vi "CALCULADORA SIRSA.vi"() -> ()   [LabVIEW 2018]
panel:
  out "accion":bool
  out "años n":dbl
  out "Actividad Actual":dbl
  out "Tiempo actual":timestamp
  in  "CONTROL":enum32{"NEUTRONES", "GAMMAS"}(tab)
  out "DISTANCIA OBTENIDA N":dbl
  out "DISTANCIA OBTENIDA N2":dbl
  in  "VALOR A CALCULAR  N":dbl
  in  "VALOR A CALCULAR  N2":dbl
  out "DISTANCIA OBTENIDA 3":dbl
  out "DISTANCIA OBTENIDA C 3":dbl
  in  "B3    3":bool
  in  "B2    3":bool
  in  "B1   3":bool
  out "DISTANCIA OBTENIDA C 2":dbl
  in  "B3    2":bool
  in  "B2    2":bool
  in  "B1   2":bool
  out "DISTANCIA OBTENIDA 2":dbl
  out "DISTANCIA OBTENIDA C":dbl
  in  "B3":bool
  in  "B2":bool
  in  "B1":bool
  out "DISTANCIA OBTENIDA":dbl
  in  "VALOR A CALCULAR":dbl
  in  "VALOR A CALCULAR  2":dbl
  in  "VALOR A CALCULAR  3":dbl
  out "Intensidad actual":dbl
  out "años":dbl
  in  "stop":bool
  # "CALCULO DE DISTANCIAS PARA UNA INTENSIDAD DE RADIACIÓN DADA"
  # "ACTIVIDAD ACTUAL"
  # "mCi"
  # "INTENSIDAD\n DESEADA EN\n     m rem/h"
  # "INTENSIDAD\n DESEADA EN\n     uSv/h"
  # "m rem/h"
  # "uSv/h"
  # "DISTANCIA CALCULADA"
  # "Distancia obtenida\npara m rem/h"
  # "Distancia obtenida\npara uSv/h"
  # "cm"
  # "cm"
  # "INTENSIDAD\n DESEADA EN\n     mR/h"
  # "INTENSIDAD\n DESEADA EN\n     uSv/h"
  # "INTENSIDAD\n DESEADA EN\n     m rem/h"
  # "mR/h"
  # "uSv/h"
  # "m rem/h"
  # "DISTANCIA CALCULADA"
  # "Distancia obtenida\npara mR/h"
  # "cm"
  # "Distancia obtenida\npara uSv/h"
  # "cm"
  # "Distancia obtenida\npara m rem/h"
  # "cm"
  # "Distancia obtenida\ncon combinacion de \nobturadores seleccionados"
  # "Distancia obtenida\ncon combinacion de \nobturadores seleccionados"
  # "Distancia obtenida\ncon combinacion de \nobturadores seleccionados"
  # "cm"
  # "cm"
  # "cm"
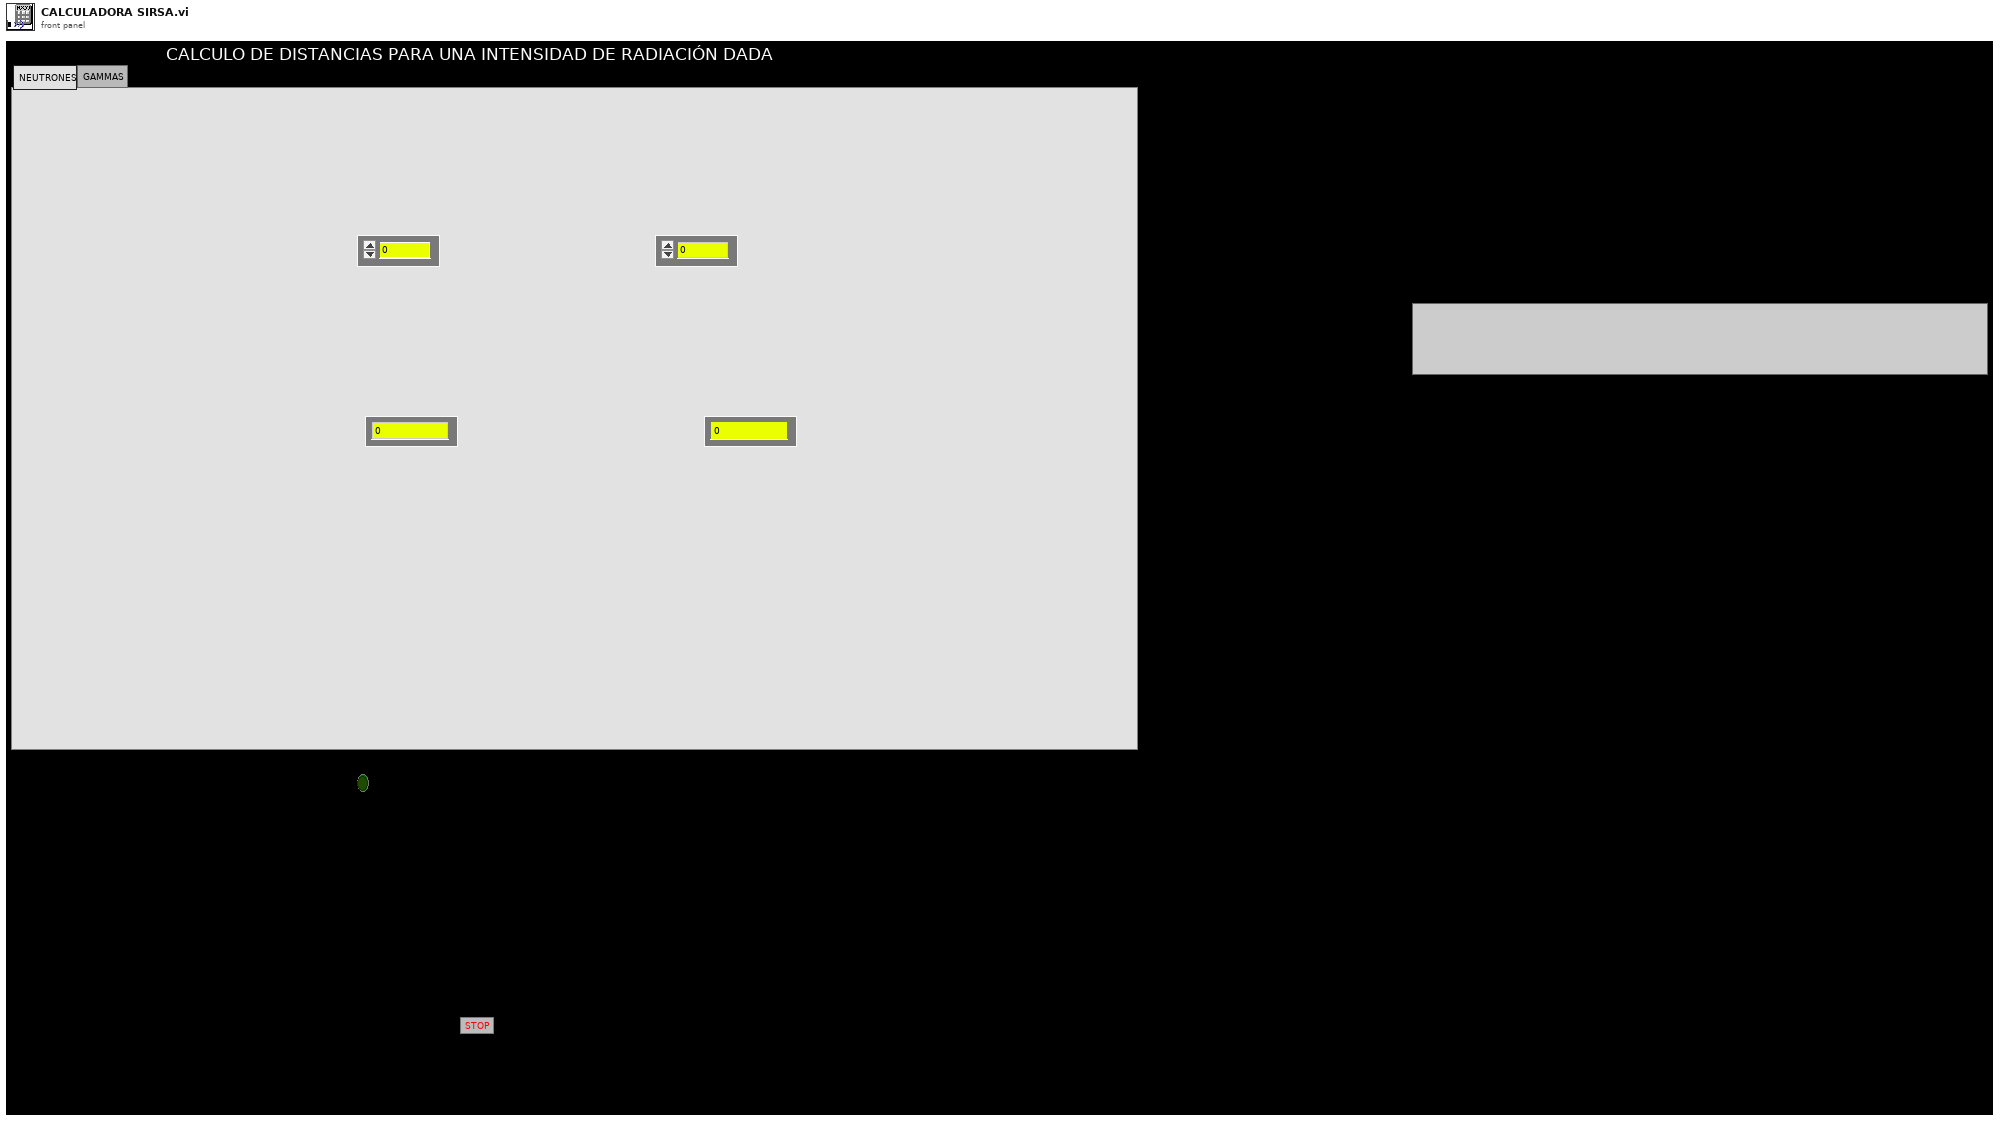
[diagram p1: front panel]
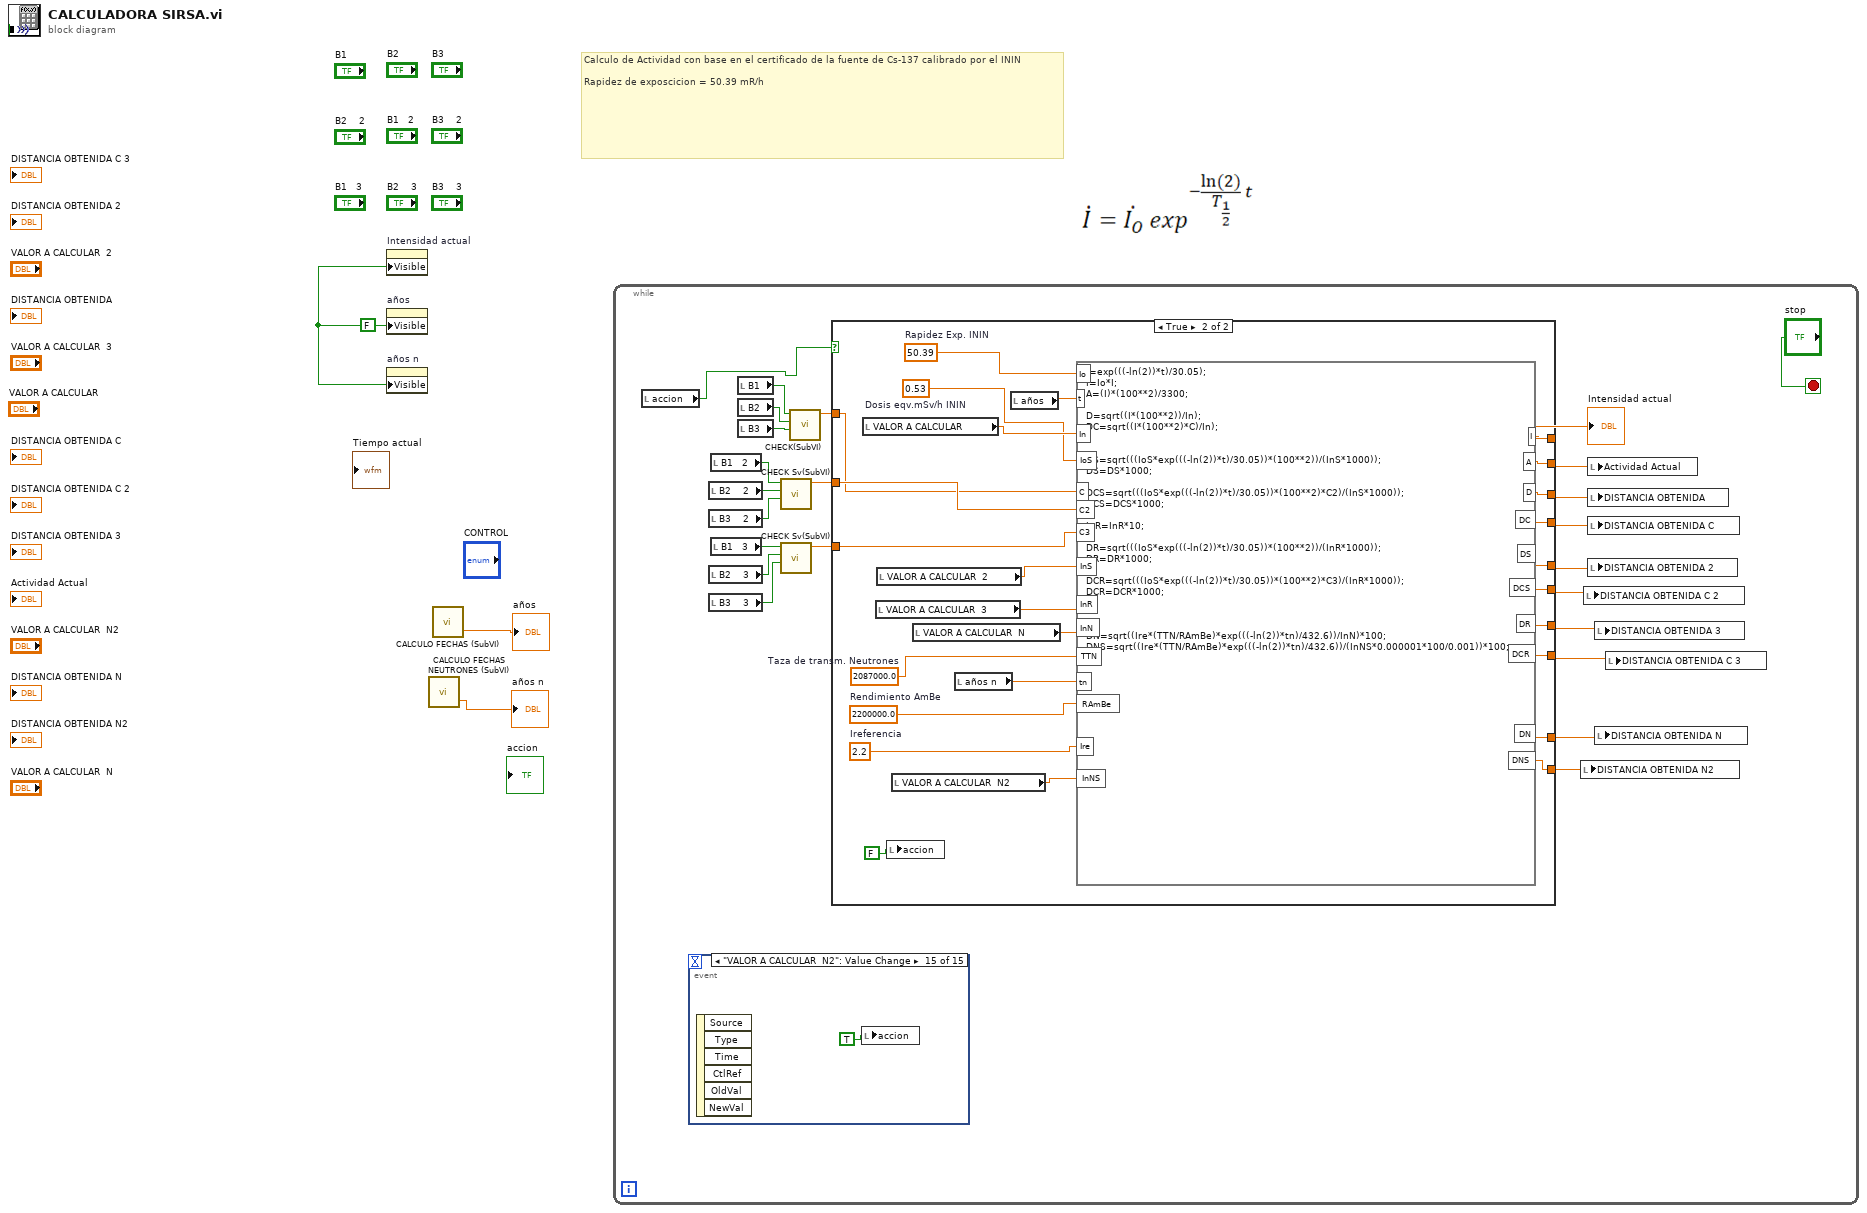
[diagram p0: block diagram]
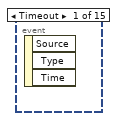
[diagram p2: hidden frame]
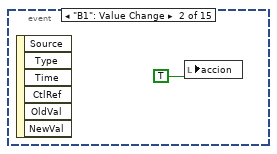
[diagram p3: hidden frame]
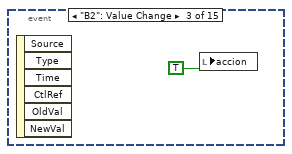
[diagram p4: hidden frame]
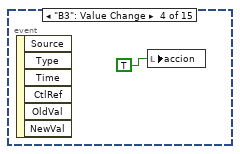
[diagram p5: hidden frame]
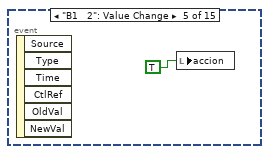
[diagram p6: hidden frame]
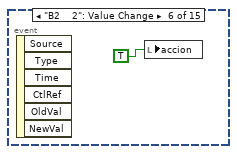
[diagram p7: hidden frame]
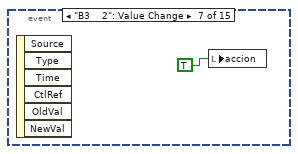
[diagram p8: hidden frame]
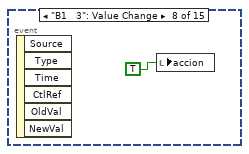
[diagram p9: hidden frame]
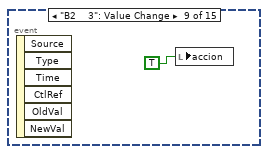
[diagram p10: hidden frame]
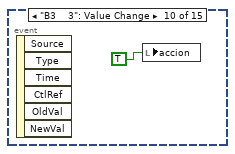
[diagram p11: hidden frame]
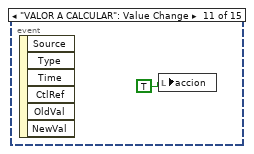
[diagram p12: hidden frame]
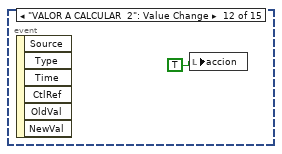
[diagram p13: hidden frame]
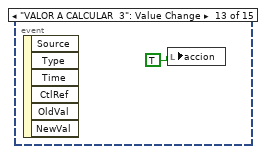
[diagram p14: hidden frame]
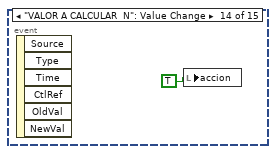
[diagram p15: hidden frame]
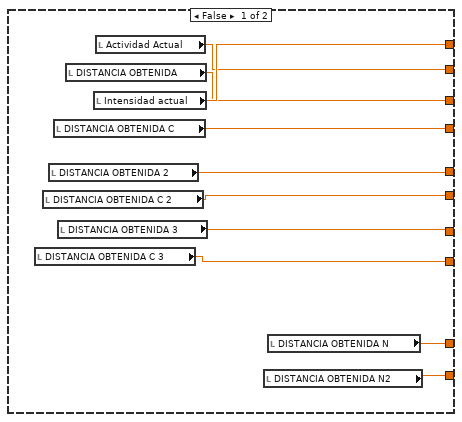
[diagram p16: hidden frame]
diagram:
  w1 = FALSE
  # "Calculo de Actividad con base en el certificado de la fuente de Cs-137 calibrado por el ININ\n\nRapidez de exposcicion = 50.39 mR/h"
  n1 = property on="Intensidad actual" class="DigNum (strict)"("Visible"=w1) -> ()  [unwired: 2 in, 2 out]
  n2 = property on="años" class="DigNum (strict)"("Visible"=w1) -> ()  [unwired: 2 in, 2 out]
  n3 = property on="años n" class="DigNum (strict)"("Visible"=w1) -> ()  [unwired: 2 in, 2 out]
  n4 = call "CALCULO FECHAS NEUTRONES (SubVI).vi"() -> ("años"=→"años n":dbl)  [unwired: 1 in, 1 out]
  n5 = call "CALCULO FECHAS (SubVI).vi"() -> ("años"=→"años":dbl)  [unwired: 1 in, 1 out]
  n6 = while {
    stop <- "stop" stop-if-true
    n7 = local read "accion"() -> (w4:bool)
    n8 = event shown="[14] \"VALOR A CALCULAR  N2\": Value Change" {
      selector: _ -> [_ _ _ _ _ _ _ _ _ _ _ _ _ _ _]
      dyn-events: _ -> [_ _ _ _ _ _ _ _ _ _ _ _ _ _ _]
      timeout: _ -> [_ _ _ _ _ _ _ _ _ _ _ _ _ _ _]
      event Timeout {
        n9 = event-data() -> ()  [unwired: 1 in, 3 out]
      }
      event "B1": Value Change {
        n10 = event-data() -> ()  [unwired: 1 in, 6 out]
        n11 = local write "accion"(TRUE) -> ()
      }
      event "B2": Value Change {
        n12 = event-data() -> ()  [unwired: 1 in, 6 out]
        n13 = local write "accion"(TRUE) -> ()
      }
      event "B3": Value Change {
        n14 = event-data() -> ()  [unwired: 1 in, 6 out]
        n15 = local write "accion"(TRUE) -> ()
      }
      event "B1   2": Value Change {
        n16 = event-data() -> ()  [unwired: 1 in, 6 out]
        n17 = local write "accion"(TRUE) -> ()
      }
      event "B2    2": Value Change {
        n18 = event-data() -> ()  [unwired: 1 in, 6 out]
        n19 = local write "accion"(TRUE) -> ()
      }
      event "B3    2": Value Change {
        n20 = event-data() -> ()  [unwired: 1 in, 6 out]
        n21 = local write "accion"(TRUE) -> ()
      }
      event "B1   3": Value Change {
        n22 = event-data() -> ()  [unwired: 1 in, 6 out]
        n23 = local write "accion"(TRUE) -> ()
      }
      event "B2    3": Value Change {
        n24 = event-data() -> ()  [unwired: 1 in, 6 out]
        n25 = local write "accion"(TRUE) -> ()
      }
      event "B3    3": Value Change {
        n26 = event-data() -> ()  [unwired: 1 in, 6 out]
        n27 = local write "accion"(TRUE) -> ()
      }
      event "VALOR A CALCULAR": Value Change {
        n28 = event-data() -> ()  [unwired: 1 in, 6 out]
        n29 = local write "accion"(TRUE) -> ()
      }
      event "VALOR A CALCULAR  2": Value Change {
        n30 = event-data() -> ()  [unwired: 1 in, 6 out]
        n31 = local write "accion"(TRUE) -> ()
      }
      event "VALOR A CALCULAR  3": Value Change {
        n32 = event-data() -> ()  [unwired: 1 in, 6 out]
        n33 = local write "accion"(TRUE) -> ()
      }
      event "VALOR A CALCULAR  N": Value Change {
        n34 = event-data() -> ()  [unwired: 1 in, 6 out]
        n35 = local write "accion"(TRUE) -> ()
      }
      event "VALOR A CALCULAR  N2": Value Change {
        n36 = event-data() -> ()  [unwired: 1 in, 6 out]
        n37 = local write "accion"(TRUE) -> ()
      }
    }
    n38 = local read "B2    2"() -> (w17:bool)
    n39 = local read "B3    2"() -> (w18:bool)
    n40 = local read "B2    3"() -> (w14:bool)
    n41 = local read "B3    3"() -> (w13:bool)
    n42 = local read "B1   2"() -> (w16:bool)
    n43 = local read "B1   3"() -> (w15:bool)
    n44 = local read "B1"() -> (w21:bool)
    n45 = local read "B2"() -> (w20:bool)
    n46 = local read "B3"() -> (w19:bool)
    n47 = call "CHECK Sv(SubVI).vi"("B3    in"=w18, "B2    in"=w17, "B1   in"=w16) -> ("Numeric"=w12:dbl)  [unwired: 8 in]
    n48 = call "CHECK Sv(SubVI).vi"("B3    in"=w13, "B2    in"=w14, "B1   in"=w15) -> ("Numeric"=w11:dbl)  [unwired: 8 in]
    n49 = call "CHECK(SubVI).vi"("B3    in"=w19, "B2    in"=w20, "B1   in"=w21) -> ("Numeric"=w22:dbl)  [unwired: 8 in]
    n50 = case shown="True" w4 {
      tunnel: [w51 w77] -> w26
      tunnel: [w50 w75] -> w25
      tunnel: [w49 w73] -> w24
      tunnel: [w48 w71] -> w23
      tunnel: w22 -> [_ w68]
      tunnel: w12 -> [_ w70]
      tunnel: w11 -> [_ w69]
      tunnel: [w47 w66] -> w10
      tunnel: [w46 w64] -> w9
      tunnel: [w45 w62] -> w8
      tunnel: [w44 w61] -> w7
      tunnel: [w43 w56] -> w6
      tunnel: [w42 w55] -> w5
      frame False {
        n51 = local read "DISTANCIA OBTENIDA C 3"() -> (w45:dbl)
        n52 = local read "DISTANCIA OBTENIDA C 2"() -> (w46:dbl)
        n53 = local read "DISTANCIA OBTENIDA 2"() -> (w47:dbl)
        n54 = local read "DISTANCIA OBTENIDA C"() -> (w48:dbl)
        n55 = local read "DISTANCIA OBTENIDA 3"() -> (w44:dbl)
        n56 = local read "DISTANCIA OBTENIDA"() -> (w49:dbl)
        n57 = local read "Intensidad actual"() -> (w51:dbl)
        n58 = local read "Actividad Actual"() -> (w50:dbl)
        n59 = local read "DISTANCIA OBTENIDA N2"() -> (w42:dbl)
        n60 = local read "DISTANCIA OBTENIDA N"() -> (w43:dbl)
      }
      frame True {
        w58 = 2.2  # Ireferencia
        w59 = 2200000.0  # Rendimiento AmBe
        w60 = 2087000.0  # Taza de transm. Neutrones
        w67 = 0.53  # Dosis eqv.mSv/h ININ
        w74 = 50.39  # Rapidez Exp. ININ
        n61 = local read "VALOR A CALCULAR"() -> (w72:dbl)
        n62 = local read "VALOR A CALCULAR  3"() -> (w63:dbl)
        n63 = local read "VALOR A CALCULAR  2"() -> (w65:dbl)
        n64 = local write "accion"(FALSE) -> ()
        n65 = local read "VALOR A CALCULAR  N2"() -> (w54:dbl)
        n66 = local read "VALOR A CALCULAR  N"() -> (w57:dbl)
        n67 = local read "años n"() -> (w53:dbl)
        n68 = local read "años"() -> (w76:dbl)
        n69 = formula code="I=exp(((-ln(2))*t)/30.05);\nI=Io*I;\nA=(I)*(100**2)/3300;\n\nD=sqrt((I*(100**2))/In);\nDC=sqrt((I*(100**2)*C)/In);\n\n\nDS=sqrt(((IoS*exp(((-ln(2))*t)/30.05))*(100**2))/(InS*1000));\nDS=DS*1000;\n\nDCS=sqrt(((IoS*exp(((-ln(2))*t)/30.05))*(100**2)*C2)/(InS*1000));\nDCS=DCS*1000;\n\nInR=InR*10;\n\nDR=sqrt(((IoS*exp(((-ln(2))*t)/30.05))*(100**2))/(InR*1000));\nDR=DR*1000;\n\nDCR=sqrt(((IoS*exp(((-ln(2))*t)/30.05))*(100**2)*C3)/(InR*1000));\nDCR=DCR*1000;\n\n\n\nDN=sqrt((Ire*(TTN/RAmBe)*exp(((-ln(2))*tn)/432.6))/InN)*100;\nDNS=sqrt((Ire*(TTN/RAmBe)*exp(((-ln(2))*tn)/432.6))/(InNS*0.000001*100/0.001))*100;"("t"=w76, "Io"=w74, "In"=w72, "C"=w68, "C2"=w70, "C3"=w69, "IoS"=w67, "InS"=w65, "InR"=w63, "TTN"=w60, "RAmBe"=w59, "Ire"=w58, "InN"=w57, "InNS"=w54, "tn"=w53) -> ("I"=w77:dbl, "A"=w75:dbl, "D"=w73:dbl, "DC"=w71:dbl, "DS"=w66:dbl, "DCS"=w64:dbl, "DCR"=w62:dbl, "DR"=w61:dbl, "DN"=w56:dbl, "DNS"=w55:dbl)
      }
    }
    "Intensidad actual" <- w26
    n70 = local write "DISTANCIA OBTENIDA N2"(w5) -> ()
    n71 = local write "DISTANCIA OBTENIDA C 2"(w9) -> ()
    n72 = local write "Actividad Actual"(w25) -> ()
    n73 = local write "DISTANCIA OBTENIDA"(w24) -> ()
    n74 = local write "DISTANCIA OBTENIDA C"(w23) -> ()
    n75 = local write "DISTANCIA OBTENIDA 2"(w10) -> ()
    n76 = local write "DISTANCIA OBTENIDA 3"(w7) -> ()
    n77 = local write "DISTANCIA OBTENIDA N"(w6) -> ()
    n78 = local write "DISTANCIA OBTENIDA C 3"(w8) -> ()
  }
